vi "AG34980A_Configure_AC_Voltage.vi"(0 "VISA resource name":refnum<visa-resource-name>, 5 "Range (5:Auto)":T2(ring)=enum."Auto", 9 "Bandwidth (1:20 Hz)":T1(ring)=enum."20 Hz", 11 "error in (no error)":errorcluster) -> (4 "VISA resource name out":refnum<visa-resource-name>, 15 "error out":errorcluster)   [LabVIEW 2022 SP3, in "DMM_Keysight_34980A.lvlib" / "DMM_Keysight_34980A.lvclass"]
doc: "This VI allows you to control the range and bandwidth settings for performing AC voltage measurements."
uses:
  DMM_Keysight_34980A.lvclass
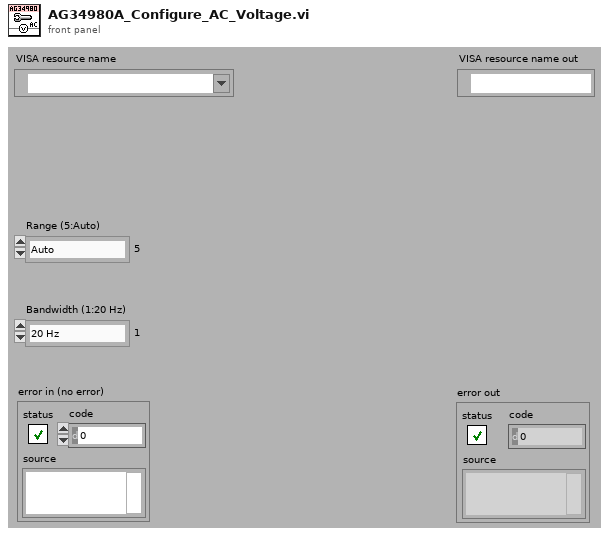
[diagram p1: front panel]
types:
  T1 = enum16{"3 Hz", "20 Hz", "200 Hz", "Minimum", "Maximum"}
  T2 = enum16{"100 mV", "1 V", "10 V", "100 V", "300 V", "Auto", "Minimum", "Maximum", "Default"}
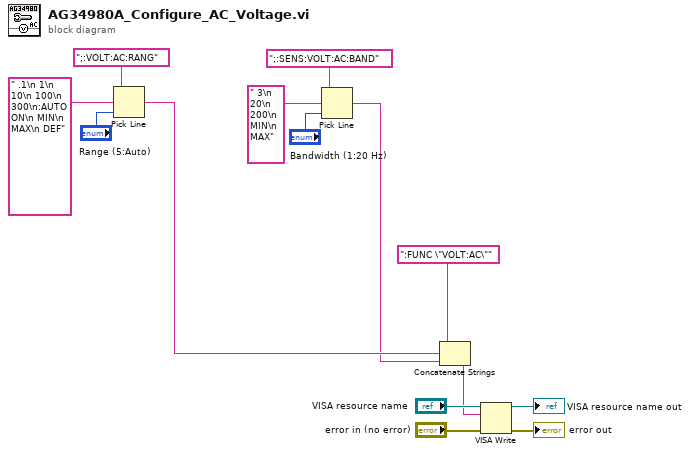
[diagram p0: block diagram]
diagram:
  n1 = Pick Line(string ("")=";:VOLT:AC:RANG", multi-line string=" .1\n 1\n 10\n 100\n 300\n:AUTO ON\n MIN\n MAX\n DEF", line index="Range (5:Auto)") -> (output string=w2:string)
  n2 = Pick Line(string ("")=";:SENS:VOLT:AC:BAND", multi-line string=" 3\n 20\n 200\n MIN\n MAX", line index="Bandwidth (1:20 Hz)") -> (output string=w1:string)
  n3 = Concatenate Strings(":FUNC \"VOLT:AC\"", w2, w1) -> (w4:string)
  n4 = VISA Write(VISA resource name="VISA resource name", write buffer=w4, error in (no error)="error in (no error)") -> (VISA resource name out=→"VISA resource name out":refnum<visa-resource-name>, error out=→"error out":errorcluster)  [unwired: 1 out]
